vi "数组比较.vi"() -> ()   [LabVIEW 2020]
doc: "本VI是为《我和LabVIEW》一书编写的示例。\n关于本书的介绍请参考网页：\nhttp://ruanqizhen.spaces.live.com/blog/cns!5852D4F797C53FB6!4310.entry"
panel:
  out "结果值":bool
  out "结果数组":bool[](array[boolean])
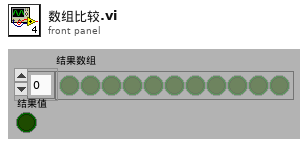
[diagram p1: front panel]
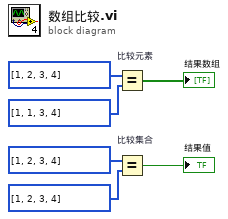
[diagram p0: block diagram]
diagram:
  n1 = Equal? "比较元素"(x=i32[] [1, 2, 3, 4], y=i32[] [1, 1, 3, 4]) -> (x = y?=→"结果数组":bool[])
  n2 = Equal? "比较集合"(x=i32[] [1, 2, 3, 4], y=i32[] [1, 2, 3, 4]) -> (x = y?=→"结果值":bool)
